vi "S2DS_Update X Y channel to scan parmeters.vi"(10 "Write channel info in":T2, 11 "Sweep info in":T1 {"Y data taking" items=["in both direction", "in up direction only", "in down direction only"]; "X data taking" items=["in both direction", "in up direction only", "in down direction only"]}) -> (2 "Write channel parameters (out)":dbl[][](array[numeric]), 3 "Sweep info out":T1 {"Y data taking" items=["in both direction", "in up direction only", "in down direction only"]; "X data taking" items=["in both direction", "in up direction only", "in down direction only"]})   [LabVIEW 2025]
uses:
  TYPE DEFS/S2DS_WC info.ctl
  TYPE DEFS/S2DS_Single WC info.ctl
  TYPE DEFS/S2DS_Sweep Info.ctl
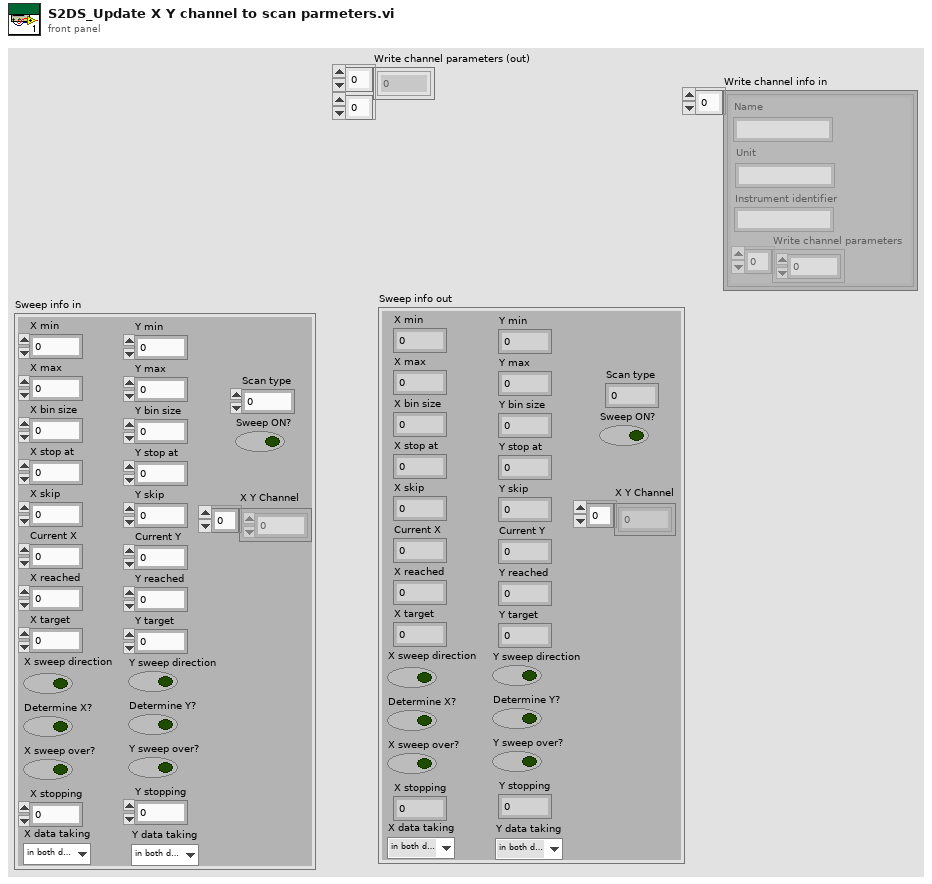
[diagram p1: front panel]
types:
  T1 = typedef "S2DS_Sweep Info.ctl" = cluster{"X min":ext, "X max":dbl, "Y min":dbl, "Y max":dbl, "X bin size":dbl, "Y bin size":dbl, "X stop at":dbl, "Y stop at":dbl, "X skip":u64, "Y skip":u64, "Current X":dbl, "Current Y":dbl, "X reached":i32, "Y reached":i32, "X target":dbl, "Y target":dbl, "Sweep ON?":bool, "X sweep direction":bool, "Y sweep direction":bool, "Determine X?":bool, "Determine Y?":bool, "X sweep over?":bool, "Y sweep over?":bool, "Scan type":i32, "X stopping":i32, "Y stopping":i32, "X Y Channel":u16[], "X data taking":u16, "Y data taking":u16}
  T2 = typedef "S2DS_WC info.ctl" = T3[]
  T3 = typedef "S2DS_Single WC info.ctl" = cluster{"Instrument identifier":string, "Write channel parameters":dbl[], "Name":string, "Unit":string}
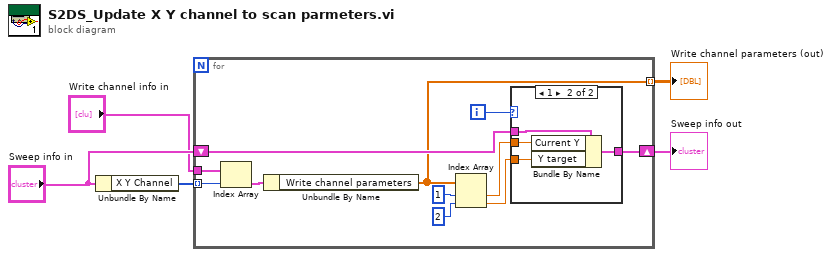
[diagram p0: block diagram]
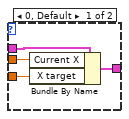
[diagram p2: hidden frame]
diagram:
  n1 = Unbundle By Name("Sweep info in") -> ("X Y Channel"=w2:u16[])
  n2 = for {
    tunnel: w2 -> [w7] mode=indexing
    shift-right: [w10] -> w4
    shift-left: "Sweep info in" -> [w13]
    tunnel: [w9] -> w5 mode=indexing
    tunnel: "Write channel info in" -> [w8]
    i -> [w14]
    n3 = Index Array(array=w8, index=w7) -> (element=w6:T3)
    n4 = Unbundle By Name(w6) -> ("Write channel parameters"=w9:dbl[])
    n5 = Index Array(array=w9, index #1=1 ("index"), index #2=2 ("index")) -> (element #1=w12:dbl, element #2=w11:dbl)
    n6 = case shown="1" w14 {
      tunnel: w13 -> [w20 w24]
      tunnel: w12 -> [w19 w22]
      tunnel: w11 -> [w18 w21]
      tunnel: [w17 w23] -> w10
      frame 0, Default {
        n7 = Bundle By Name(cluster=w20, "Current X"=w19, "X target"=w18) -> (w17:T1)
      }
      frame 1 {
        n8 = Bundle By Name(cluster=w24, "Current Y"=w22, "Y target"=w21) -> (w23:T1)
      }
    }
  }
  "Write channel parameters (out)" <- w5
  "Sweep info out" <- w4
